vi "Priority.vi"(8 "error in (no error)":errorcluster, 11 "PathValidation in":refnum<class "PathValidation.lvclass">) -> (0 "error out":errorcluster, 2 "Priority":u16, 3 "PathValidation out":refnum<class "PathValidation.lvclass">)   [LabVIEW 2020, in "HTTP Server.lvlib" / "PathValidation.lvclass"]
uses:
  PathValidation.lvclass
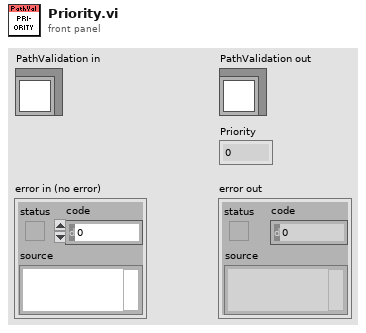
[diagram p1: front panel]
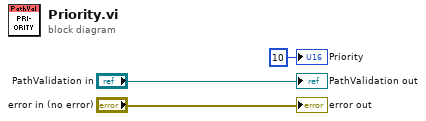
[diagram p0: block diagram]
diagram:
  "error out" <- "error in (no error)"
  "PathValidation out" <- "PathValidation in"
  "Priority" <- u16 10 ("Priority")
